vi "5-parameter-stanford-response -- analytic derivatives -- grad and curvature -- V6.vi"(7 "action":T2=enum."onlygrads", 8 "parameters map  IN":map{T1, dbl}(c390), 10 "ω (rad/sec)":dbl=0.1 format="%#_10f") -> (0 "parameters map  OUT":map{T1, dbl}(c390), 1 "λdζ(ω)/dλ OUT":map{T1, cdb}(c390), 2 "ω out (rad/sec)":dbl=0.1 format="%#_10f", 3 "ζ(ω) OUT":cdb=0.1+0.0i format="%#_10f")   [LabVIEW 2021]
uses:
  3-lorentzian-heat-response action.ctl
  3-lorentzian-parameters.ctl
panel:
  in  "κ0":dbl(slide)=6.091279771876994e-09 min=0.0 max=0.3 step=1e-12 scale=1e-10..1e-06 scale format="%#_3p"
  in  "ζ":dbl(slide)=0.016395386176563286 min=0.0 max=0.3 step=1e-06 scale=1e-05..1000.0 scale format="%#_3p"
  in  "τN":dbl(slide)=0.0007964886373917906 min=0.0 max=0.3 step=1e-06 scale=1e-06..10.0 scale format="%#_3p"
  in  "T1":dbl(slide)=0.017784241145719432 min=0.0 max=0.3 step=1e-06 scale=0.0001..10.0 scale format="%#_3p"
  in  "τC":dbl(slide)=0.0055481925503790405 min=0.0 max=0.3 step=1e-06 scale=0.0001..10.0 scale format="%#_3p"
  in  "τS":dbl(slide)=0.01833817297436167 min=0.0 max=0.3 step=1e-06 scale=0.0001..10.0 scale format="%#_3p"
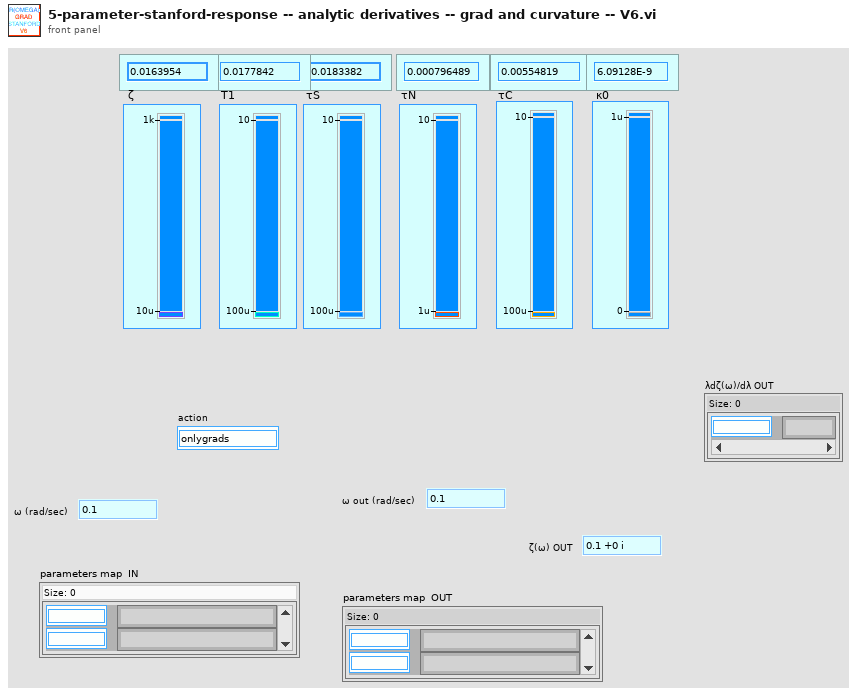
[diagram p1: front panel]
types:
  T1 = typedef "3-lorentzian-parameters.ctl" = enum16{"ζ", "τ1", "τS", "τN", "τC", "κ0", "m1", "m2", "m3", "T (K)", "B (T)", "θ (deg)", "side (S|R)", "set of (B|T)", "Re(offset)", "Im(offset)", "στ1", "στ1-", "στ1+", "στS", "στS-", "στS+", "στN", "στN-", "στN+", "τ11", "τ12", "τ21", "τ22", "τN1", "τN2", "σηlogτ1", "σηlogτS", "σηlogτN", "σlogτ1", "σlogτS", "σlogτN", "σητ1", "σητS", "σητN", "noiseT", "plain", "vproj"}
  T2 = typedef "3-lorentzian-heat-response action.ctl" = enum16{"calc R", "create string", "calc m1m2m3", "dζ", "dT1", "dτS", "dτN", "dτC", "d-all", "dκ0", "T(K)", "m1", "m2", "m3", "parse string", "θ (deg)", "B (T)", "onlygrads", "newton", "create emty string", "simple2nd", "calc R2", "ScalarProd", "ScalarProd-diff", "nothing", "ScalarProd-eta", "tolog", "ignore", "three2nd", "eta-errors"}
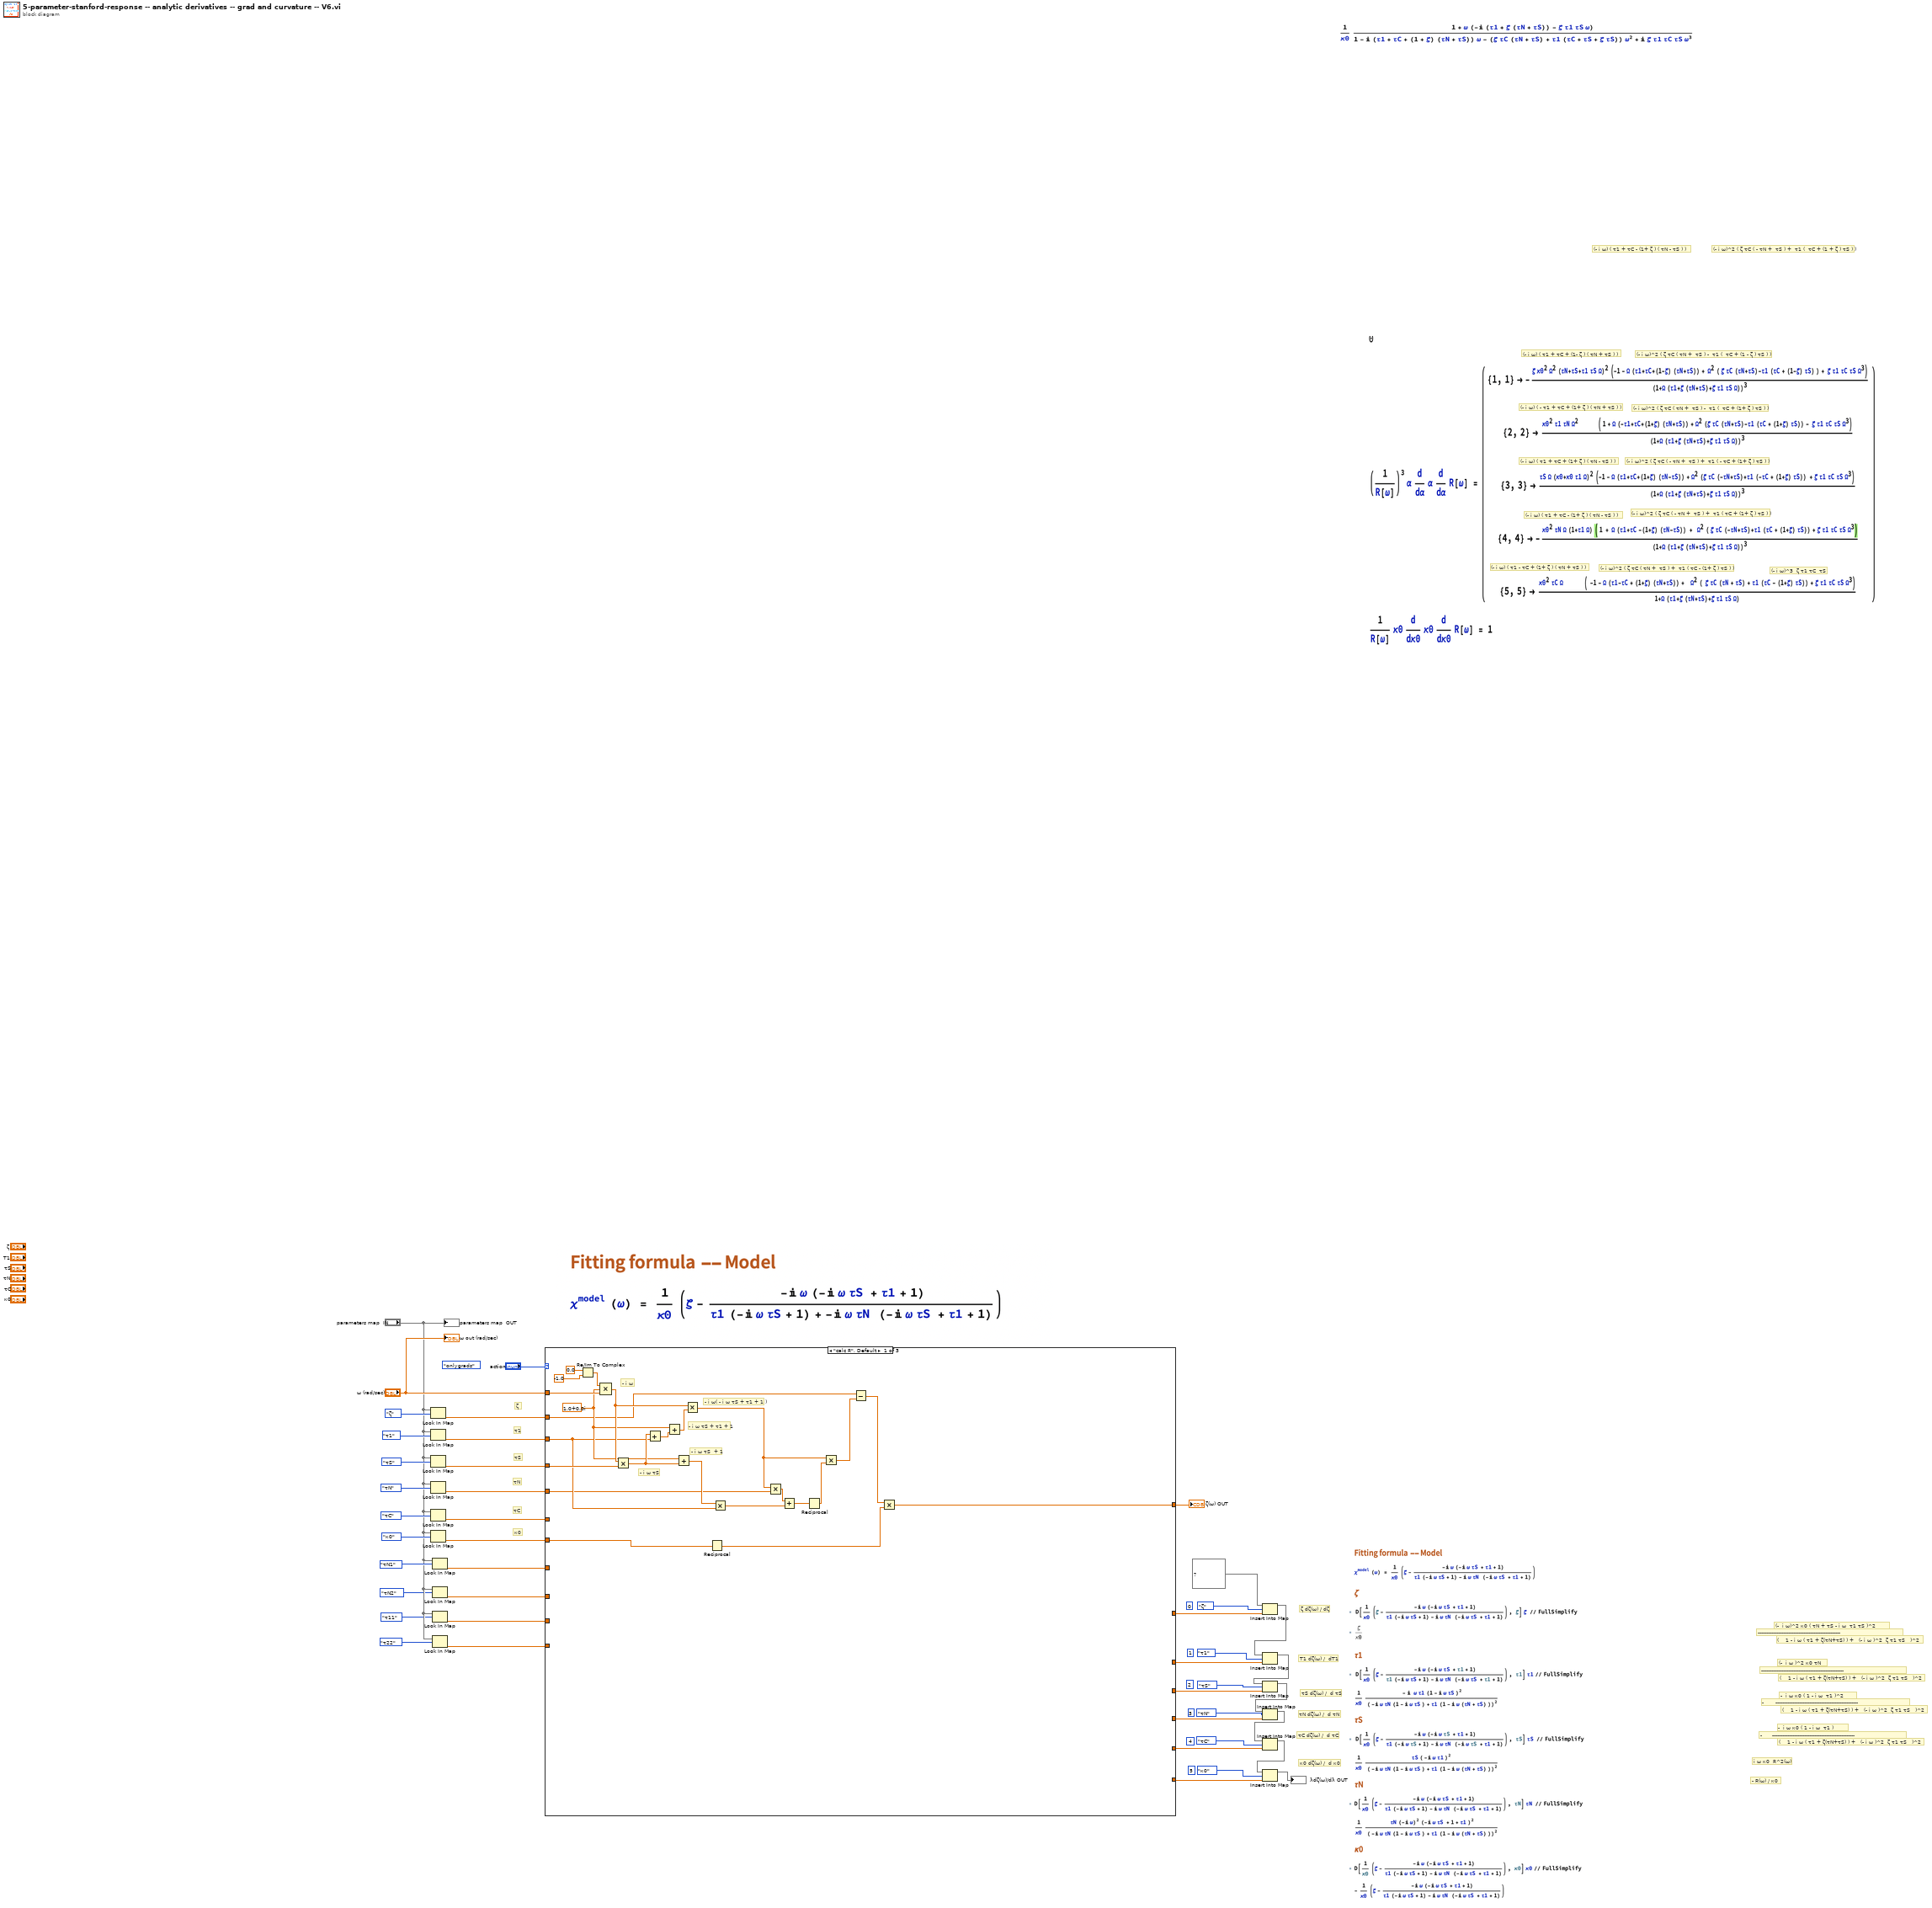
[diagram p0: block diagram]
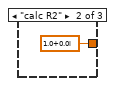
[diagram p2: hidden frame]
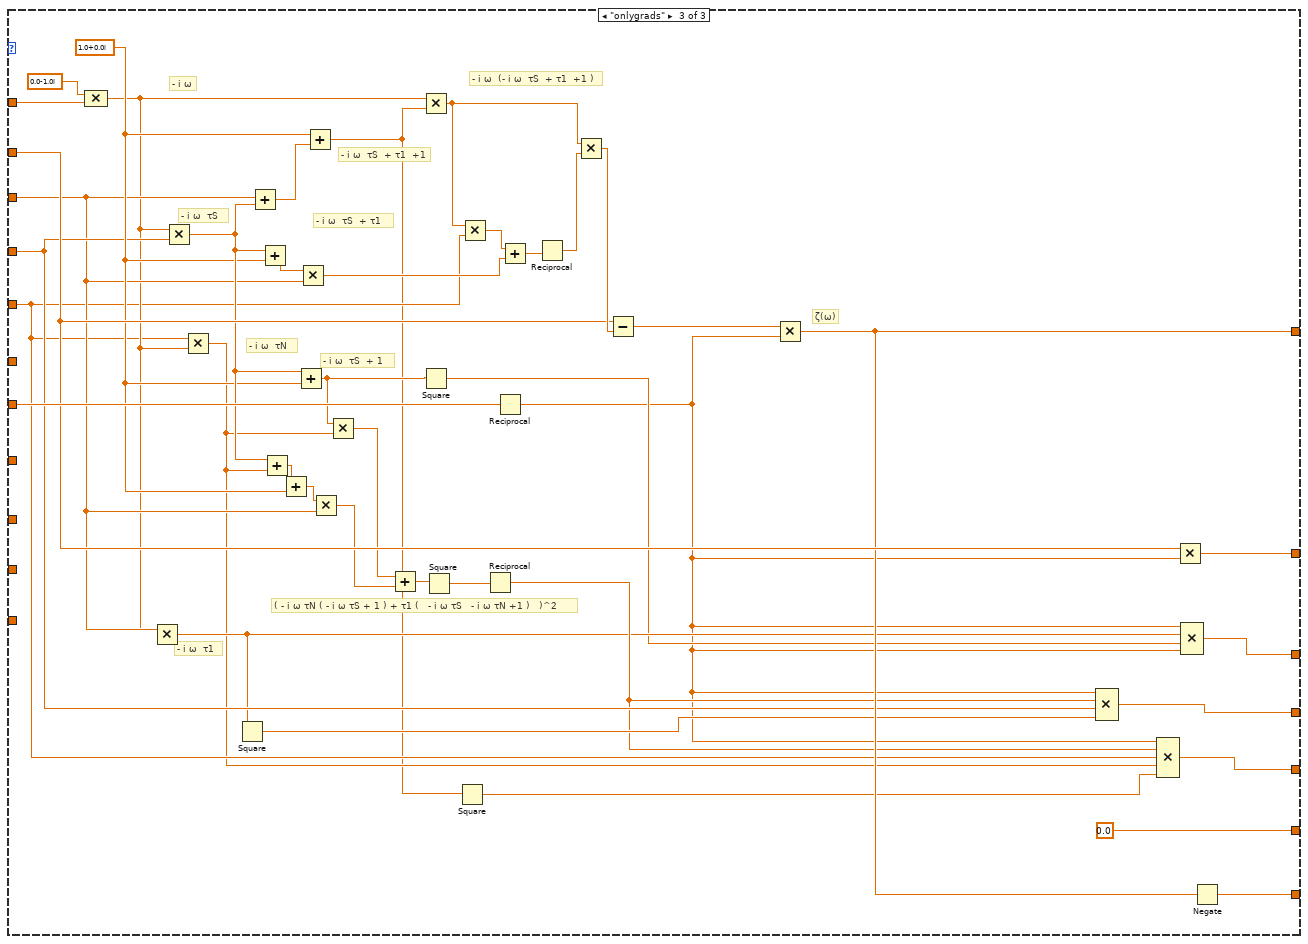
[diagram p3: hidden frame]
diagram:
  (unwired) 3-lorentzian-heat-response_action."onlygrads" ("action")
  (unwired) 5 ("key")
  (unwired) 4 ("key")
  (unwired) 3 ("key")
  (unwired) 2 ("key")
  (unwired) 1 ("key")
  (unwired) 0 ("key")
  # "-------------------------------------------------"
  # "(-  i ω)^2 κ0 ( τN + τS - i ω  τ1 τS )^2"
  # "(    1 - i ω ( τ1 + ζ(τN+τS) ) +   (- i ω )^2  ζ τ1 τS   )^2"
  # "-------------------------------------------------"
  # "(-  i ω )^2 κ0 τN"
  # "(    1 - i ω ( τ1 + ζ(τN+τS) ) +   (- i ω )^2  ζ τ1 τS   )^2"
  # "-      -------------------------------------------------"
  # "-  i ω κ0 ( 1 - i ω  τ1 )"
  # "(    1 - i ω ( τ1 + ζ(τN+τS) ) +   (- i ω )^2  ζ τ1 τS   )^2"
  # "-       -------------------------------------------------"
  # "-  i ω κ0 ( 1 - i ω  τ1 )^2"
  # "(    1 - i ω ( τ1 + ζ(τN+τS) ) +   (- i ω )^2  ζ τ1 τS   )^2"
  # "i ω κ0  R^2(ω)"
  # "- R(ω) / κ0"
  # "κ0 dζ(ω) /  d κ0"
  # "τC dζ(ω) /  d τC"
  # "τN dζ(ω) /  d τN"
  # "τS dζ(ω) /  d τS"
  # "T1 dζ(ω) /  dT1"
  # "ζ dζ(ω) / dζ"
  # "(- i ω)^2 ( ζ τC ( - τN +  τS ) +  τ1 (  τC + (1 + ζ ) τS ) )"
  # "(- i ω) ( τ1 + τC - (1+ ζ ) ( τN - τS ) )"
  # "(- i ω)^2 ( ζ τC ( τN +  τS ) -  τ1 (  τC + (1 - ζ ) τS ) )"
  # "(- i ω) ( τ1 + τC + (1- ζ ) ( τN + τS ) )"
  # "(- i ω)^2 ( ζ τC ( τN +  τS ) -  τ1 (  τC + (1+ ζ ) τS ) )"
  # "(- i ω) ( - τ1 + τC + (1+ ζ ) ( τN + τS ) )"
  # "(- i ω)^2 ( ζ τC ( - τN +  τS ) +  τ1 ( - τC + (1+ ζ ) τS ) )"
  # "(- i ω) ( τ1 + τC + (1+ ζ ) ( τN - τS ) )"
  # "(- i ω)^2 ( ζ τC ( - τN +  τS ) +  τ1 ( τC + (1+ ζ ) τS ) )"
  # "(- i ω) ( τ1 + τC - (1+ ζ ) ( τN - τS ) )"
  # "(- i ω)^3  ζ τ1 τC  τS"
  # "(- i ω) ( τ1 - τC + (1+ ζ ) ( τN + τS ) )"
  # "(- i ω)^2 ( ζ τC ( τN +  τS ) +  τ1 ( τC - (1+ ζ ) τS ) )"
  # "κ0"
  # "τC"
  # "τN"
  # "τS"
  # "τ1"
  # "ζ"
  n1 = Look In Map(map="parameters map  IN", key=3-lorentzian-parameters."ζ" ("Plost: sweep window")) -> (value=w35:dbl)  [unwired: 1 in, 1 out]
  n2 = Look In Map(map="parameters map  IN", key=3-lorentzian-parameters."τ1" ("Plost: sweep window")) -> (value=w34:dbl)  [unwired: 1 in, 1 out]
  n3 = Look In Map(map="parameters map  IN", key=3-lorentzian-parameters."τS" ("Plost: sweep window")) -> (value=w33:dbl)  [unwired: 1 in, 1 out]
  n4 = Look In Map(map="parameters map  IN", key=3-lorentzian-parameters."τN" ("Plost: sweep window")) -> (value=w32:dbl)  [unwired: 1 in, 1 out]
  n5 = Look In Map(map="parameters map  IN", key=3-lorentzian-parameters."τC" ("Plost: sweep window")) -> (value=w31:dbl)  [unwired: 1 in, 1 out]
  n6 = Look In Map(map="parameters map  IN", key=3-lorentzian-parameters."κ0" ("Plost: sweep window")) -> (value=w30:dbl)  [unwired: 1 in, 1 out]
  n7 = Look In Map(map="parameters map  IN", key=3-lorentzian-parameters."τN1" ("Plost: sweep window")) -> (value=w3:dbl)  [unwired: 1 in, 1 out]
  n8 = Look In Map(map="parameters map  IN", key=3-lorentzian-parameters."τN2" ("Plost: sweep window")) -> (value=w2:dbl)  [unwired: 1 in, 1 out]
  n9 = Look In Map(map="parameters map  IN", key=3-lorentzian-parameters."τ11" ("Plost: sweep window")) -> (value=w4:dbl)  [unwired: 1 in, 1 out]
  n10 = Look In Map(map="parameters map  IN", key=3-lorentzian-parameters."τ22" ("Plost: sweep window")) -> (value=w1:dbl)  [unwired: 1 in, 1 out]
  n11 = case shown="\"calc R\", Default" "action" {
    tunnel: w31 -> [_ _ _]
    tunnel: "ω (rad/sec)" -> [w64 _ w109]
    tunnel: w34 -> [w56 _ w80]
    tunnel: w32 -> [w55 _ w72]
    tunnel: w33 -> [w63 _ w81]
    tunnel: w35 -> [w49 _ w94]
    tunnel: [w44 cdb 1.0+0.0i w92] -> w43
    tunnel: w30 -> [w47 _ w104]
    tunnel: [_ _ w91] -> w20
    tunnel: [_ _ 0.0] -> w22
    tunnel: [_ _ w108] -> w25
    tunnel: [_ _ w107] -> w24
    tunnel: [_ _ w106] -> w27
    tunnel: [_ _ w93] -> w29
    tunnel: w4 -> [_ _ _]
    tunnel: w3 -> [_ _ _]
    tunnel: w2 -> [_ _ _]
    tunnel: w1 -> [_ _ _]
    frame "calc R", Default {
      w58 = cdb 1.0+0.0i ("value")
      # "- i ω τS  + 1"
      # "- i ω( - i ω τS + τ1 + 1 )"
      # "- i ω τS + τ1 + 1"
      # "- i ω τS"
      # "- i ω"
      n12 = Re/Im To Complex(1:-1.0 ("y"), 2:0.0 ("x")) -> (0:w65:cdb)
      n13 = Compound Arithmetic op=MULTIPLY(w65, w58, w64) -> (w60:cdb)
      n14 = Multiply(x=w60, y=w63) -> (x*y=w59:cdb)
      n15 = Add(x=w59, y=w56) -> (x+y=w62:cdb)
      n16 = Add(x=w58, y=w62) -> (x+y=w61:cdb)
      n17 = Add(x=w58, y=w59) -> (x+y=w57:cdb)
      n18 = Multiply(x=w60, y=w61) -> (x*y=w51:cdb)
      n19 = Reciprocal(x=w47) -> (1/x=w45:dbl)
      n20 = Multiply(x=w57, y=w56) -> (x*y=w53:cdb)
      n21 = Multiply(x=w51, y=w55) -> (x*y=w54:cdb)
      n22 = Add(x=w54, y=w53) -> (x+y=w52:cdb)
      n23 = Reciprocal(x=w52) -> (1/x=w50:cdb)
      n24 = Multiply(x=w51, y=w50) -> (x*y=w48:cdb)
      n25 = Subtract(x=w49, y=w48) -> (x-y=w46:cdb)
      n26 = Multiply(x=w46, y=w45) -> (x*y=w44:cdb)
    }
    frame "calc R2" {
    }
    frame "onlygrads" {
      w86 = cdb 1.0+0.0i ("value")
      # "- i ω  τ1"
      # "- i ω  τS  + 1"
      # "- i ω  τN"
      # "( - i ω τN ( - i ω τS + 1 ) + τ1 (   - i ω τS   - i ω τN +1 )   )^2"
      # "ζ(ω)"
      # "- i ω  (- i ω  τS  + τ1  +1 )"
      # "- i ω  τS  + τ1  +1"
      # "- i ω  τS  + τ1"
      # "- i ω  τS"
      # "- i ω"
      n27 = Compound Arithmetic op=MULTIPLY(cdb 0.0-1.0i ("value"), w109) -> (w79:cdb)
      n28 = Multiply(x=w80, y=w79) -> (x*y=w76:cdb)
      n29 = Multiply(x=w79, y=w81) -> (x*y=w87:cdb)
      n30 = Multiply(x=w72, y=w79) -> (x*y=w71:cdb)
      n31 = Square(x=w76) -> (x^2=w78:cdb)
      n32 = Add(x=w80, y=w87) -> (x+y=w103:cdb)
      n33 = Add(x=w87, y=w86) -> (x+y=w102:cdb)
      n34 = Add(x=w87, y=w71) -> (x+y=w89:cdb)
      n35 = Add(x=w89, y=w86) -> (x+y=w88:cdb)
      n36 = Add(x=w87, y=w86) -> (x+y=w75:cdb)
      n37 = Multiply(x=w102, y=w80) -> (x*y=w100:cdb)
      n38 = Add(x=w86, y=w103) -> (x+y=w70:cdb)
      n39 = Multiply(x=w88, y=w80) -> (x*y=w84:cdb)
      n40 = Multiply(x=w75, y=w71) -> (x*y=w85:cdb)
      n41 = Add(x=w85, y=w84) -> (x+y=w83:cdb)
      n42 = Multiply(x=w79, y=w70) -> (x*y=w98:cdb)
      n43 = Square(x=w75) -> (x^2=w74:cdb)
      n44 = Square(x=w83) -> (x^2=w82:cdb)
      n45 = Square(x=w70) -> (x^2=w69:cdb)
      n46 = Multiply(x=w98, y=w72) -> (x*y=w101:cdb)
      n47 = Reciprocal(x=w82) -> (1/x=w77:cdb)
      n48 = Reciprocal(x=w104) -> (1/x=w73:dbl)
      n49 = Add(x=w101, y=w100) -> (x+y=w99:cdb)
      n50 = Reciprocal(x=w99) -> (1/x=w97:cdb)
      n51 = Multiply(x=w98, y=w97) -> (x*y=w96:cdb)
      n52 = Subtract(x=w94, y=w96) -> (x-y=w95:cdb)
      n53 = Multiply(x=w95, y=w73) -> (x*y=w92:cdb)
      n54 = Compound Arithmetic op=MULTIPLY(w73, w77, w81, w78) -> (w108:cdb)
      n55 = Compound Arithmetic op=MULTIPLY(w73, w77, w72, w71, w69) -> (w107:cdb)
      n56 = Multiply(x=w94, y=w73) -> (x*y=w93:dbl)
      n57 = Compound Arithmetic op=MULTIPLY(w73, w76, w74, w73) -> (w106:cdb)
      n58 = Negate(x=w92) -> (-x=w91:cdb)
    }
  }
  "ζ(ω) OUT" <- w43
  n59 = Insert Into Map(map in=map{T1, cdb} {} ("parameters map  IN 2"), key=3-lorentzian-parameters."ζ" ("Plost: sweep window"), value=w29) -> (map out=w28:map{T1, cdb})  [unwired: 2 out]
  n60 = Insert Into Map(map in=w28, key=3-lorentzian-parameters."τ1" ("Plost: sweep window"), value=w27) -> (map out=w26:map{T1, cdb})  [unwired: 2 out]
  n61 = Insert Into Map(map in=w26, key=3-lorentzian-parameters."τS" ("Plost: sweep window"), value=w25) -> (map out=w19:map{T1, cdb})  [unwired: 2 out]
  n62 = Insert Into Map(map in=w19, key=3-lorentzian-parameters."τN" ("Plost: sweep window"), value=w24) -> (map out=w23:map{T1, cdb})  [unwired: 2 out]
  n63 = Insert Into Map(map in=w23, key=3-lorentzian-parameters."τC" ("Plost: sweep window"), value=w22) -> (map out=w21:map{T1, cdb})  [unwired: 2 out]
  n64 = Insert Into Map(map in=w21, key=3-lorentzian-parameters."κ0" ("Plost: sweep window"), value=w20) -> (map out=→"λdζ(ω)/dλ OUT":map{T1, cdb})  [unwired: 2 out]
  "ω out (rad/sec)" <- "ω (rad/sec)"
  "parameters map  OUT" <- "parameters map  IN"
